vi "ni5660 Sub Multi-Span Concatenation.vi"(0 "FFT spectrum array":cluster{"f0":dbl, "df":dbl, "spectrum":cdb[]}[](array[cluster]) {"spectrum" format="%.2f"; "df" format="%.2f"; "f0" format="%.2f"}, 2 "Fstart":dbl format="%.2f", 3 "Fstop":dbl format="%.2f", 5 "spectral info in":T2, 11 "error in (no error)":errorcluster) -> (4 "concatenated FFT spectrum":cluster{"f0":dbl, "df":dbl, "spectrum":cdb[]} {"spectrum" format="%.2f"; "df" format="%.2f"; "f0" format="%.2f"}, 6 "spectral info out":T1={"spectrum type"=enum."Power [Magnitude^2]", "linear/dB"=enum."linear", "window"=0, "window size"=1024, "FFT size"=1024} {"window" items=["None ", "Hanning", "Hamming", "Blackman-Harris", "Exact Blackman", "Blackman", "Flat Top", "4 Term B-Harris ", "7 Term B-Harris", "Low Sidelobe"]}, 14 "data ready?":bool, 15 "error out":errorcluster)   [LabVIEW 2011]
doc: "This example acquires and computes an averaged power spectrum across a frequency range wider than 20 MHz. The frequency range is defined by <B>Fstart</B> and <B>Fstop</B>. You can control the averaging type applied to the spectrum, the units in which to return the spectrum and the size of each data segment. This VI is a sub-VI of the RFSA Multi-Span Application VI."
uses:
  <vilib>/measure/masml.llb/ma_sml_Spectral Info.ctl
  <vilib>/Analysis/1siggen.llb/Ramp Pattern by Samples.vi
  <vilib>/addons/Spectral Measurements Toolset/LVSupport/SMT Examples Utilities/smt_ Overlap Arrays(real).vi
  <vilib>/addons/Spectral Measurements Toolset/LVSupport/SMT Examples Utilities/smt_ Overlap Arrays(complex).vi
  <vilib>/Analysis/NI_AALBase.lvlib
  <vilib>/measure/NI_MAPro.lvlib
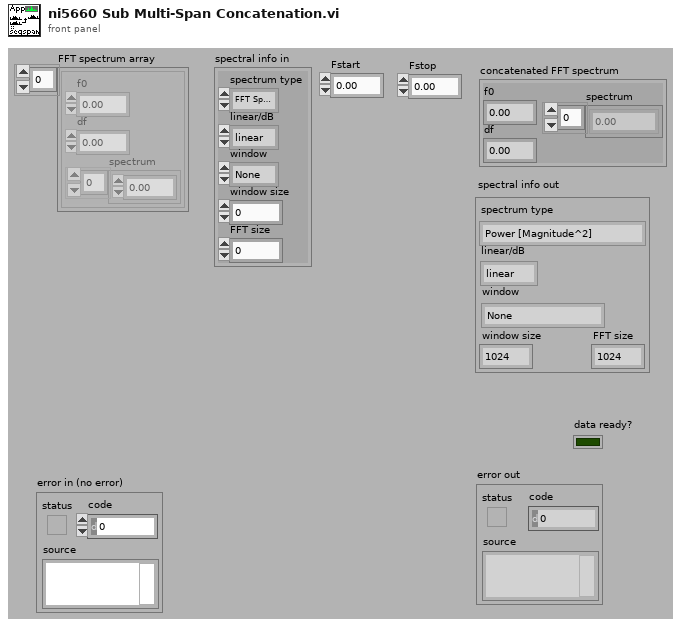
[diagram p1: front panel]
types:
  T1 = typedef "NI_MAPro.lvlib/ma_sml_Spectral Info.ctl" = cluster{"spectrum type":enum16{"FFT Spectrum [complex]", "Amplitude [Magnitude]", "Power [Magnitude^2]", "Cross Spectrum [complex]", "Frequency Response [Complex]"}, "linear/dB":enum16{"linear", "dB"}, "window":u16, "window size":i32, "FFT size":i32}
  T2 = cluster{"spectrum type":enum16{"FFT Spectrum [complex]", "Amplitude [Magnitude]", "Power [Magnitude^2]", "Cross Spectrum [complex]", "Frequency Response [Complex]"}, "linear/dB":enum16{"linear", "dB"}, "window":enum16{"None ", "Hanning", "Hamming", "Blackman-Harris", "Exact Blackman", "Blackman", "Flat Top", "4 Term B-Harris ", "7 Term B-Harris", "Low Sidelobe"}, "window size":i32, "FFT size":i32}
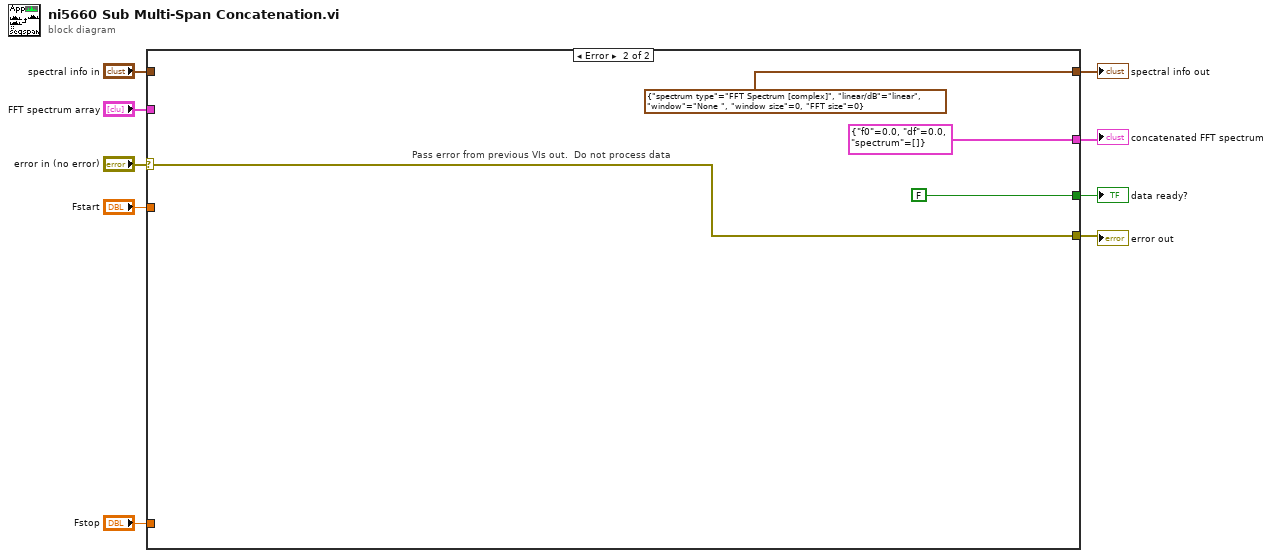
[diagram p0: block diagram]
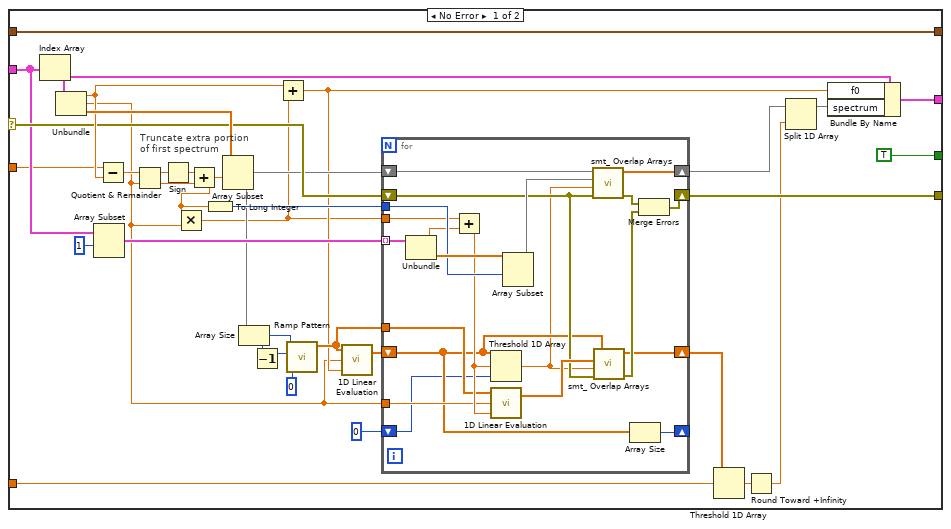
[diagram p2: hidden frame]
diagram:
  n1 = case shown="Error" "error in (no error)" {
    selector: "error in (no error)" -> [w34 w68]
    tunnel: [w33 w68] -> w9
    tunnel: "FFT spectrum array" -> [w15 _]
    tunnel: "Fstart" -> [w14 _]
    tunnel: "Fstop" -> [w13 _]
    tunnel: [w10 cluster{"f0":dbl, "df":dbl, "spectrum":cdb[]} {"f0"=0.0, "df"=0.0, "spectrum"=[]}] -> w1
    tunnel: [w11 T2 {"spectrum type"=enum."FFT Spectrum [complex]", "linear/dB"=enum."linear", "window"=enum."None ", "window size"=0, "FFT size"=0} ("spectral info in")] -> w4
    tunnel: [TRUE ("data ready?") FALSE ("data ready?")] -> w3
    tunnel: "spectral info in" -> [w11 _]
    frame No Error {
      # "Truncate extra portion\nof first spectrum"
      n2 = Index Array(array=w15) -> (element=w43:cluster{"f0":dbl, "df":dbl, "spectrum":cdb[]})  [unwired: 1 in]
      n3 = Unbundle(w43) -> ("f0"=w35:dbl, "df"=w19:dbl, "spectrum"=w39:cdb[])
      n4 = Array Subset(array=w15, index=1 ("Array Index")) -> (w37:cluster{"f0":dbl, "df":dbl, "spectrum":cdb[]}[])  [unwired: 1 in]
      n5 = Subtract(x=w14, y=w35) -> (x-y=w42:dbl)
      n6 = Quotient & Remainder(x=w42, y=w19) -> (x-y*floor(x/y)=w41:dbl, floor(x/y)=w18:dbl)
      n7 = Sign(1:w41) -> (0:w40:dbl)
      n8 = Add(x=w40, y=w18) -> (x+y=w20:dbl)
      n9 = Multiply(x=w20, y=w19) -> (x*y=w16:dbl)
      n10 = To Long Integer(number=w20) -> (32bit integer=w36:i32)
      n11 = Array Subset(array=w39, index=w20) -> (w32:cdb[])  [unwired: 1 in]
      n12 = Array Size(array=w32) -> (size(s)=w30:i32)
      n13 = Decrement(x=w30) -> (x-1=w17:i32)
      n14 = Add(x=w35, y=w16) -> (x+y=w28:dbl)
      n15 = call-poly <vilib>:"Ramp Pattern.vi"("start"=0, "end"=w17, "samples"=w30) -> ("Ramp Pattern"=w29:dbl[])  [unwired: 7 in, 1 out]
      n16 = call <vilib>:"1D Linear Evaluation.vi"("offset"=w28, "scale"=w19, "X"=w29) -> ("Y[i]=X[i]*a+b"=w27:dbl[])  [unwired: 1 out]
      n17 = for {
        shift-right: [w52] -> w23
        shift-left: w32 -> [w61]
        shift-right: [w48] -> w24
        shift-left: w27 -> [w47]
        tunnel: w37 -> [w64] mode=indexing
        tunnel: w36 -> [w62]
        tunnel: w16 -> [w59]
        shift-right: [w49] -> w33
        shift-left: w34 -> [w53]
        shift-right: [w46] -> _
        shift-left: 0 -> [w45]
        tunnel: w19 -> [w55]
        tunnel: w29 -> [w54]
        n18 = Unbundle(w64) -> ("f0"=w58:dbl, "spectrum"=w63:cdb[])  [unwired: 1 out]
        n19 = Add(x=w59, y=w58) -> (x+y=w56:dbl)
        n20 = Threshold 1D Array(1:w45, 2:w56, 3:w47) -> (0:w44:dbl)
        n21 = call <vilib>:"1D Linear Evaluation.vi"("offset"=w56, "scale"=w55, "X"=w54) -> ("Y[i]=X[i]*a+b"=w57:dbl[])  [unwired: 1 out]
        n22 = Array Subset(array=w63, index=w62) -> (w60:cdb[])  [unwired: 1 in]
        n23 = call-poly <vilib>:"smt_ Overlap Arrays.vi"("error in (no error)"=w53, "start index"=w44, "Array 2"=w60, "Array 1"=w61) -> ("error out"=w51:errorcluster, "Array Out"=w52:cdb[])  [unwired: 2 in]
        n24 = call-poly <vilib>:"smt_ Overlap Arrays.vi"("error in (no error)"=w53, "start index"=w44, "Array 2"=w57, "Array 1"=w47) -> ("error out"=w50:errorcluster, "Array Out"=w48:dbl[])  [unwired: 2 in]
        n25 = Array Size(array=w47) -> (size(s)=w46:i32)
        n26 = Merge Errors(w51, w50) -> (w49:errorcluster)
      }
      n27 = Threshold 1D Array(2:w13, 3:w24) -> (0:w25:dbl)  [unwired: 1 in]
      n28 = Round Toward +Infinity(x=w25) -> (ceil(x): smallest int >= x=w22:dbl)
      n29 = Split 1D Array(array=w23, index=w22) -> (first subarray=w21:cdb[])  [unwired: 1 out]
      n30 = Bundle By Name(cluster=w43, "f0"=w28, "spectrum"=w21) -> (w10:cluster{"f0":dbl, "df":dbl, "spectrum":cdb[]})
    }
    frame Error {
      # "Pass error from previous VIs out.  Do not process data"
    }
  }
  "error out" <- w9
  "spectral info out" <- w4
  "data ready?" <- w3
  "concatenated FFT spectrum" <- w1
